vi "sortmeasdata_OK.vi"(1 "Array":u16[](array[numeric]), 2 "MeasData 2":T1) -> (0 "output cluster":T1)   [LabVIEW 2010]
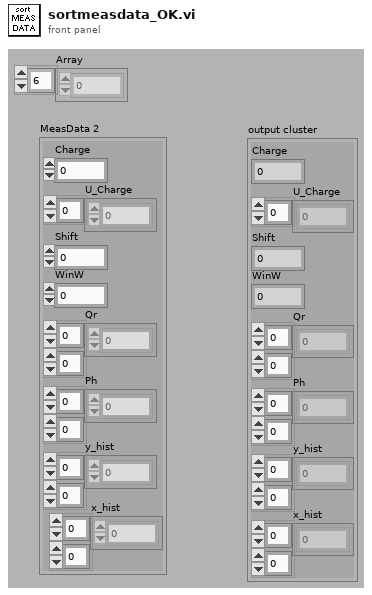
[diagram p1: front panel]
types:
  T1 = cluster{"Charge":i32, "U_Charge":i32[], "Shift":i32, "WinW":i32, "Qr":i32[][], "Ph":i32[][], "y_hist":i32[][], "x_hist":i32[][]}
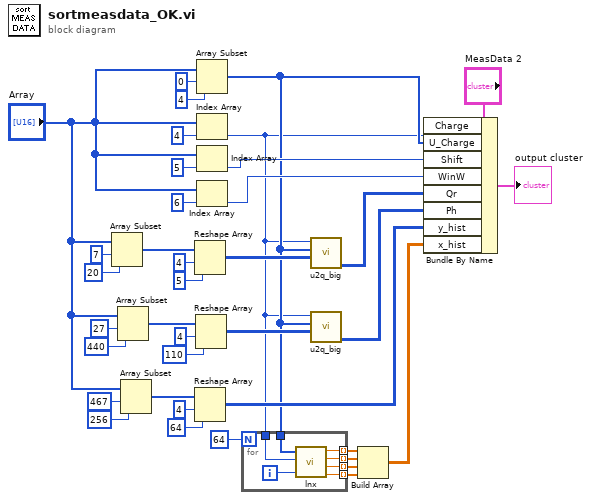
[diagram p0: block diagram]
diagram:
  n1 = Array Subset(array="Array", index=7, length=20) -> (w21:u16[])
  n2 = Array Subset(array="Array", index=27, length=440) -> (w14:u16[])
  n3 = Array Subset(array="Array", index=467, length=256) -> (w13:u16[])
  n4 = Reshape Array(w21, 4 ("dimension size"), 5 ("dimension size")) -> (w6:u16[][])
  n5 = Reshape Array(w13, 4 ("dimension size"), 64 ("dimension size")) -> (w12:u16[][])
  n6 = Reshape Array(w14, 4 ("dimension size"), 110 ("dimension size")) -> (w4:u16[][])
  n7 = Array Subset(array="Array", index=0, length=4) -> (w3:u16[])
  n8 = Index Array(array="Array", index=4) -> (element=w2:u16)
  n9 = Index Array(array="Array", index=5) -> (element=w34:u16)
  n10 = Index Array(array="Array", index=6) -> (element=w33:u16)
  n11 = for {
    N: 64 -> [_]
    tunnel: w2 -> [w45]
    tunnel: w3 -> [w44]
    tunnel: [w43] -> w10 mode=indexing
    tunnel: [w42] -> w9 mode=indexing
    tunnel: [w41] -> w8 mode=indexing
    tunnel: [w40] -> w7 mode=indexing
    i -> [w39]
    n12 = call "lnx.vi"("U_ch"=w44, "Ch"=w45, "i"=w39) -> ("x1"=w43:dbl, "x2"=w42:dbl, "x3"=w41:dbl, "x4"=w40:dbl)
  }
  n13 = call "u2q_big.vi"("In"=w6, "U_Ch"=w3, "Ch"=w2) -> ("Out"=w5:i32[][])
  n14 = call "u2q_big.vi"("In"=w4, "U_Ch"=w3, "Ch"=w2) -> ("Out"=w1:i32[][])
  n15 = Build Array(w10, w9, w8, w7) -> (w32:dbl[][])
  n16 = Bundle By Name(cluster="MeasData 2", "Charge"=w2, "U_Charge"=w3, "Shift"=w34, "WinW"=w33, "Qr"=w5, "Ph"=w1, "y_hist"=w12, "x_hist"=w32) -> (→"output cluster":T1)
